vi "HW3j&j.vi"() -> ()   [LabVIEW 2015]
panel:
  out "Numeric":i32
  in  "stop":bool
  out "error out":errorcluster
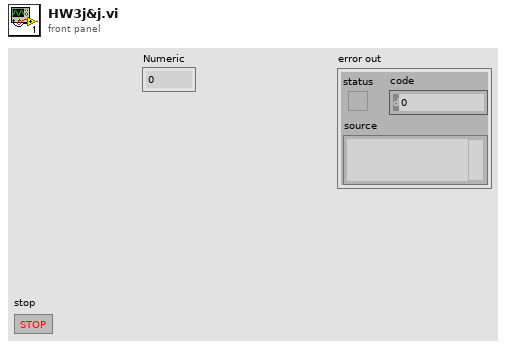
[diagram p1: front panel]
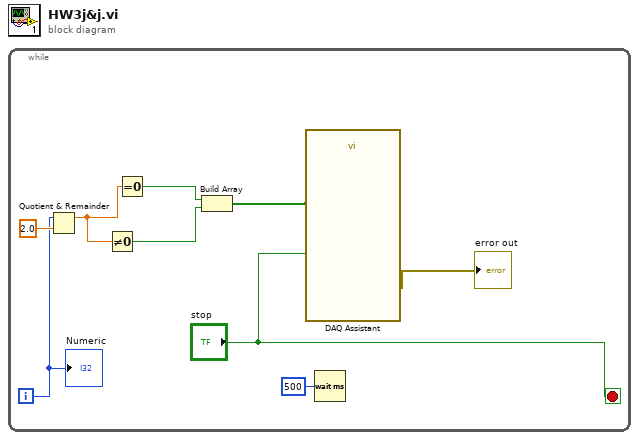
[diagram p0: block diagram]
diagram:
  n1 = while {
    i -> [w5]
    stop <- "stop" stop-if-true
    n2 = Quotient & Remainder(x=w5, y=2.0) -> (x-y*floor(x/y)=w2:dbl)  [unwired: 1 out]
    n3 = Not Equal To 0?(x=w2) -> (x != 0?=w3:bool)
    n4 = Equal To 0?(x=w2) -> (x = 0?=w7:bool)
    n5 = Build Array(w7, w3) -> (w8:bool[])
    n6 = call "DAQ Assistant"("data"=w8, "stop (T)"="stop") -> ("error out"=→"error out":errorcluster)  [unwired: 16 in, 1 out]
    n7 = Wait (ms)(milliseconds to wait=u32 500) -> ()  [unwired: 1 out]
    "Numeric" <- w5
  }
